vi "RSZVB Trace Statistical Evaluation.vi"(7 "Info Field (F: Off)":bool, 8 "error in (no error)":errorcluster {"code" format="%.0x"}, 9 "Statistical Parameter (0: All)":i32(ring) items=["All", "Mean", "Std Deviation", "Max", "Min", "RMS", "Peak-to-peak", "Electrical Length", "Phase Delay", "Slope", "Flatness", "Gain"], 10 "Channel (Trace) (1)":i32=1, 11 "VISA session":refnum<visa-resource-name>) -> (0 "error out":errorcluster {"code" format="%.0x"}, 2 "Response Value":dbl[](array[numeric]) format="%^.3e", 3 "dup VISA session":refnum<visa-resource-name>)   [LabVIEW 2011]
doc: "This VI selects how to evaluate and display statistical and phase information of the entire trace or of a specific evaluation range.\n\nRemote-control command(s):\nCALCulate<Ch/Tr>:STATistics[:STATe] <Boolean>\nCALCulate<Ch/Tr>:STATistics:RESult? MEAN | STDDev | MAX | MIN | RMS | PTPeak | ELENgth | PDELay | ALL | SLOPe | FLATness | GAIN"
panel:
  # "On\nOff"
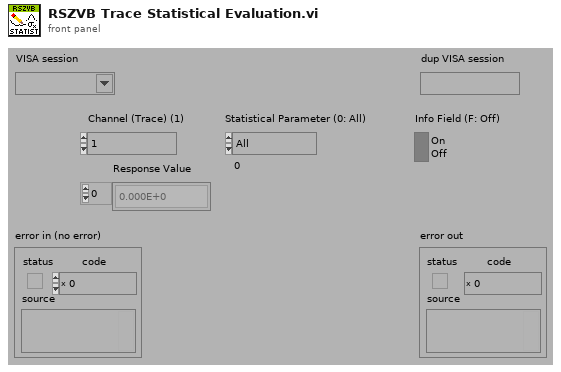
[diagram p1: front panel]
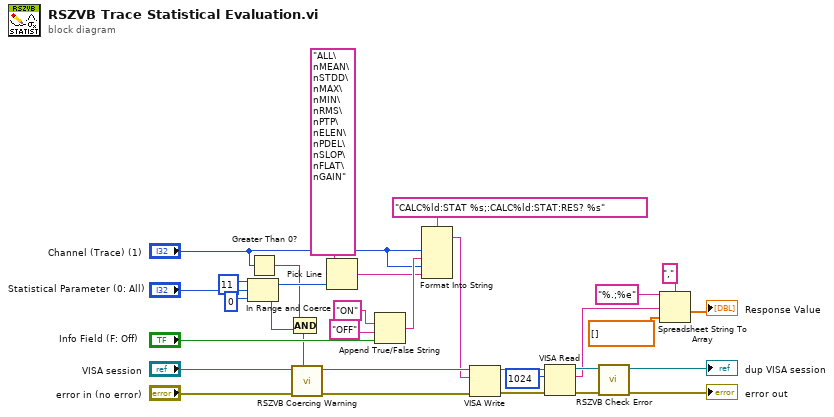
[diagram p0: block diagram]
diagram:
  n1 = In Range and Coerce(upper limit=11, x="Statistical Parameter (0: All)", lower limit=0) -> (coerced(x)=w13:i32, In Range?=w11:bool)
  n2 = Greater Than 0?(x="Channel (Trace) (1)") -> (x > 0?=w10:bool)
  n3 = Compound Arithmetic op=AND(w10, w11) -> (w12:bool)
  n4 = call "RSZVB Coercing Warning.vi"("In Range?"=w12, "error in (no error)"="error in (no error)", "VISA session"="VISA session") -> ("error out"=w28:errorcluster, "dup VISA session"=w29:refnum<visa-resource-name>)  [unwired: 7 in]
  n5 = Pick Line(multi-line string="ALL\nMEAN\nSTDD\nMAX\nMIN\nRMS\nPTP\nELEN\nPDEL\nSLOP\nFLAT\nGAIN", line index=w13) -> (output string=w8:string)  [unwired: 1 in]
  n6 = Append True/False String(1:"Info Field (F: Off)", 2:"OFF", 3:"ON") -> (0:w26:string)  [unwired: 1 in]
  n7 = Format Into String(format string="CALC%ld:STAT %s;:CALC%ld:STAT:RES? %s", "Channel (Trace) (1)", w26, "Channel (Trace) (1)", w8) -> (resulting string=w27:string)  [unwired: 2 in, 1 out]
  n8 = VISA Write(VISA resource name=w29, write buffer=w27, error in (no error)=w28) -> (VISA resource name out=w15:refnum<visa-resource-name>, error out=w17:errorcluster)  [unwired: 1 out]
  n9 = VISA Read(VISA resource name=w15, byte count=u32 1024 ("byte count (0)"), error in (no error)=w17) -> (VISA resource name out=w22:refnum<visa-resource-name>, read buffer=w6:string, error out=w21:errorcluster)  [unwired: 1 out]
  n10 = call "RSZVB Check Error.vi"("error in (no error)"=w21, "VISA session"=w22) -> ("error out"=→"error out":errorcluster, "dup VISA session"=→"dup VISA session":refnum<visa-resource-name>)  [unwired: 8 in]
  n11 = Spreadsheet String To Array(delimiter (Tab)=",", format string="%.;%e", spreadsheet string=w6, array type (2D Dbl)=dbl[] []) -> (array=→"Response Value":dbl[])
